vi "CurrentPressure.vi"() -> ()   [LabVIEW 2013]
panel:
  in  "CurrentPressure":dbl
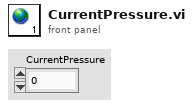
[diagram p1: front panel]
diagram:
